vi "PointerToCoordinate.vi"(8 "Return Type":T1(ring), 9 "Chunk length":u8, 10 "Voxel length":dbl, 11 "Voxel pointer":cluster{i32, i32, i32, i32, i32, i32, i32}) -> (3 "Coordinates":cluster{dbl, dbl, dbl})   [LabVIEW 2014]
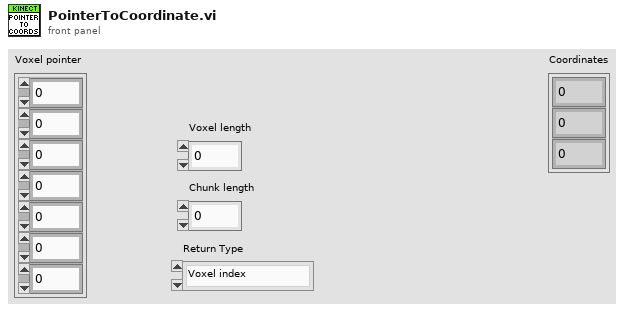
[diagram p1: front panel]
types:
  T1 = enum16{"Voxel index", "Inches", "Voxel center (in)"}
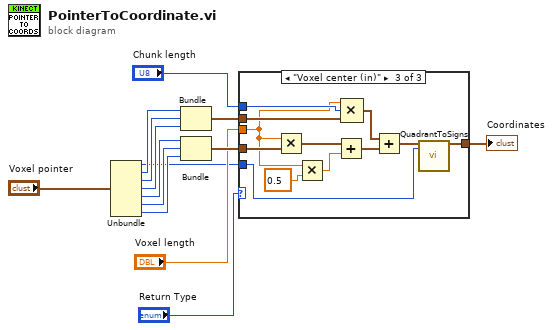
[diagram p0: block diagram]
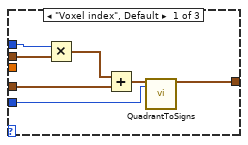
[diagram p2: hidden frame]
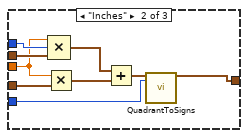
[diagram p3: hidden frame]
diagram:
  n1 = Unbundle("Voxel pointer") -> (w2:i32, w13:i32, w12:i32, w11:i32, w10:i32, w9:i32, w8:i32)
  n2 = Bundle(w13, w12, w11) -> (w6:cluster{i32, i32, i32})  [unwired: 1 in]
  n3 = Bundle(w10, w9, w8) -> (w5:cluster{i32, i32, i32})  [unwired: 1 in]
  n4 = case shown="\"Voxel center (in)\"" "Return Type" {
    tunnel: w6 -> [w20 w30 w42]
    tunnel: w5 -> [w18 w27 w39]
    tunnel: "Voxel length" -> [_ w22 w31]
    tunnel: "Chunk length" -> [w21 w29 w41]
    tunnel: w2 -> [w16 w24 w37]
    tunnel: [w15 w23 w36] -> w1
    frame "Voxel index", Default {
      n5 = Multiply(x=w21, y=w20) -> (x*y=w19:cluster{i32, i32, i32})
      n6 = Add(x=w19, y=w18) -> (x+y=w17:cluster{i32, i32, i32})
      n7 = call "QuadrantToSigns.vi"("Point"=w17, "Quadrant"=w16) -> ("Point Out"=w15:cluster{"X":sgl, "Y":sgl, "Z":sgl})  [unwired: 17 in]
    }
    frame "Inches" {
      n8 = Multiply(x=w22, y=w27) -> (x*y=w26:cluster{dbl, dbl, dbl})
      n9 = Compound Arithmetic op=MULTIPLY(w22, w29, w30) -> (w28:cluster{dbl, dbl, dbl})
      n10 = Add(x=w28, y=w26) -> (x+y=w25:cluster{dbl, dbl, dbl})
      n11 = call "QuadrantToSigns.vi"("Point"=w25, "Quadrant"=w24) -> ("Point Out"=w23:cluster{"X":sgl, "Y":sgl, "Z":sgl})  [unwired: 17 in]
    }
    frame "Voxel center (in)" {
      n12 = Multiply(x=w31, y=w39) -> (x*y=w34:cluster{dbl, dbl, dbl})
      n13 = Multiply(x=w31, y=0.5) -> (x*y=w33:dbl)
      n14 = Add(x=w34, y=w33) -> (x+y=w35:cluster{dbl, dbl, dbl})
      n15 = Compound Arithmetic op=MULTIPLY(w31, w41, w42) -> (w40:cluster{dbl, dbl, dbl})
      n16 = Add(x=w40, y=w35) -> (x+y=w38:cluster{dbl, dbl, dbl})
      n17 = call "QuadrantToSigns.vi"("Point"=w38, "Quadrant"=w37) -> ("Point Out"=w36:cluster{"X":sgl, "Y":sgl, "Z":sgl})  [unwired: 17 in]
    }
  }
  "Coordinates" <- w1
